vi "Main.vi"() -> ()   [LabVIEW 2014]
uses:
  QTMDriver 2013/CustomIO.ctl
  <vilib>/myRIO/Instrument Drivers/Onboard IO/AI/typedefs/AI Reference.ctl
  <vilib>/myRIO/Common/Instrument Driver Framework/Utilities/typedefs/myRIO Generic Hardware Reference.ctl
  <vilib>/myRIO/Common/Instrument Driver Framework/Utilities/typedefs/Hardware Version Enum.ctl
  <vilib>/myRIO/Common/Instrument Driver Framework/Utilities/typedefs/myRIO v1.0 Reference.ctl
  <vilib>/myRIO/Common/Instrument Driver Framework/Utilities/typedefs/Generic FPGA Reference.ctl
  <vilib>/myRIO/Common/Instrument Driver Framework/myRIO v1.0/AI/typedefs/AI Channels List.ctl
  <vilib>/myRIO/Common/Instrument Driver Framework/myRIO v1.0/AI/typedefs/AI Channels Enum.ctl
  <vilib>/myRIO/Common/Instrument Driver Framework/Utilities/typedefs/Analog Scaling Constants List.ctl
  <vilib>/myRIO/Common/Instrument Driver Framework/Utilities/typedefs/Analog Scaling Constants.ctl
  <vilib>/userdefined/High Color/nirio_resource_hc.ctl
  <vilib>/myRIO/Common/Instrument Driver Framework/Utilities/vis/Is FPGA Ref Available.vi
  <vilib>/myRIO/Common/Instrument Driver Framework/myRIO v1.0/AI/vis/myRIO v1.1 Open AI.vi
  <vilib>/myRIO/Instrument Drivers/Onboard IO/AI/vis/Read.vi
  <vilib>/myRIO/Common/Instrument Driver Framework/Utilities/vis/Validate Channels.vi
  <vilib>/myRIO/Common/Instrument Driver Framework/myRIO v1.0/AI/vis/myRIO v1.0 Reserve AI.vi
  <vilib>/myRIO/Common/Instrument Driver Framework/myRIO v1.0/UART/vis/myRIO v1.0 Close UART.vi
  <vilib>/myRIO/Common/Instrument Driver Framework/myRIO v1.0/AI/vis/myRIO v1.0 Build MUX Configuration AI.vi
  <vilib>/myRIO/Common/Instrument Driver Framework/myRIO v1.0/Resource Manager/vis/myRIO v1.0 Reserve Channel List.vi
  <vilib>/myRIO/Common/Instrument Driver Framework/myRIO v1.0/Resource Manager/vis/myRIO v1.0 Reserve Channel.vi
  <vilib>/myRIO/Common/Instrument Driver Framework/myRIO v1.0/Resource Manager/vis/myRIO v1.0 Unreserve Channel.vi
  <vilib>/myRIO/Common/Instrument Driver Framework/myRIO v1.0/Resource Manager/vis/myRIO v1.0 Build Mutex Name.vi
  <vilib>/Utility/VariantDataType/GetNumericInfo.vi
  <vilib>/Utility/error.llb/Error Cluster From Error Code.vi
  <vilib>/myRIO/Common/Instrument Driver Framework/myRIO v1.0/myRIO v1.1 Open.vi
  <vilib>/myRIO/Common/Instrument Driver Framework/myRIO v1.0/AI/vis/myRIO v1.0 Get Scaling Constants AI.vi
  <vilib>/myRIO/Common/Instrument Driver Framework/Utilities/vis/IO Manager.vi
  <vilib>/myRIO/Common/Instrument Driver Framework/Utilities/vis/Configuration Manager.vi
  <vilib>/myRIO/Common/Instrument Driver Framework/myRIO v1.0/myRIO v1.0 Close.vi
  <vilib>/myRIO/Common/Instrument Driver Framework/myRIO v1.0/AI/vis/myRIO v1.0 Read AI.vi
  <vilib>/myRIO/Common/Instrument Driver Framework/Utilities/vis/FPGA Ref Manager.vi
  <vilib>/myRIO/Common/Instrument Driver Framework/myRIO v1.0/myRIO v1.0 Reset FPGA.vi
  <vilib>/myRIO/Common/Instrument Driver Framework/myRIO v1.0/IRQ/vis/myRIO v1.0 IRQ Info FGV.vi
  <vilib>/myRIO/Common/Instrument Driver Framework/myRIO v1.0/IRQ/vis/myRIO v1.0 Timer IRQ Info FGV.vi
  <vilib>/myRIO/Common/Instrument Driver Framework/myRIO v1.0/IRQ/vis/myRIO v1.0 ISR Agent.vi
  <vilib>/myRIO/Express VI/Onboard IO/AI/AI Express VI.xnode
  <vilib>/myRIO/Instrument Drivers/Onboard IO/AI/vis/myRIO AI Open.xnode
  <vilib>/myRIO/Instrument Drivers/Utilities/Utilities.lvlib
  <vilib>/myRIO/Instrument Drivers/Onboard IO/AI/AI.lvlib
panel:
  out "p_d":dbl[](array[numeric])
  in  "psiplot 4":cluster{"psi_d":dbl, "psi":dbl}
  out "p_d":dbl[](array[numeric])
  out "wpPath":cluster{"x":dbl, "y":dbl}[](array[cluster])
  out "iOut WPDP":dbl
  out "psiplot WPDP":cluster{"Double":dbl, "y_r":dbl, "y":dbl}(graph)
  out "yplot WPDP":cluster{"Double":dbl, "y_r":dbl, "y":dbl}(graph)
  out "xplot WPDP":cluster{"Double":dbl, "y_r":dbl, "y":dbl}(graph)
  out "WithinProximity WPDP":bool
  out "e_psi 2":dbl
  out "45degrees":bool
  out "iOut":dbl
  out "e_psi":dbl
  out "proximity straight":dbl
  out "plotpsi str":cluster{"psi_d":dbl, "psi":dbl}(graph)
  out "psiplot str":cluster{"psi_d":dbl, "psi":dbl}
  in  "u":dbl[](array[numeric])
  out "plotdelta":dbl(graph)
  out "plotpsi":cluster{"psi_d":dbl, "psi":dbl}(graph)
  out "WithinProximity radius":bool
  out "proximity":dbl
  out "psiplot 3":cluster{"psi_d":dbl, "psi":dbl}
  out "psiplot 2":cluster{"e_d":dbl, "e_r":dbl, "psi":dbl}
  out "yplot 2":cluster{"y_d":dbl, "y_r":dbl, "y":dbl}
  out "xplot 2":cluster{"x_d":dbl, "x_r":dbl, "x":dbl}
  out "psiplot":cluster{"Double":dbl, "y_r":dbl, "y":dbl}(graph)
  out "yplot":cluster{"Double":dbl, "y_r":dbl, "y":dbl}(graph)
  out "xplot":cluster{"Double":dbl, "y_r":dbl, "y":dbl}(graph)
  out "straightPath":cluster{"x":dbl, "y":dbl}[](array[cluster])
  out "ellipsePath":cluster{"x":dbl, "y":dbl}[](array[cluster])
  out "y":dbl
  out "x":dbl
  out "B/AI2 (Pin 7)":dbl
  in  "stop":bool
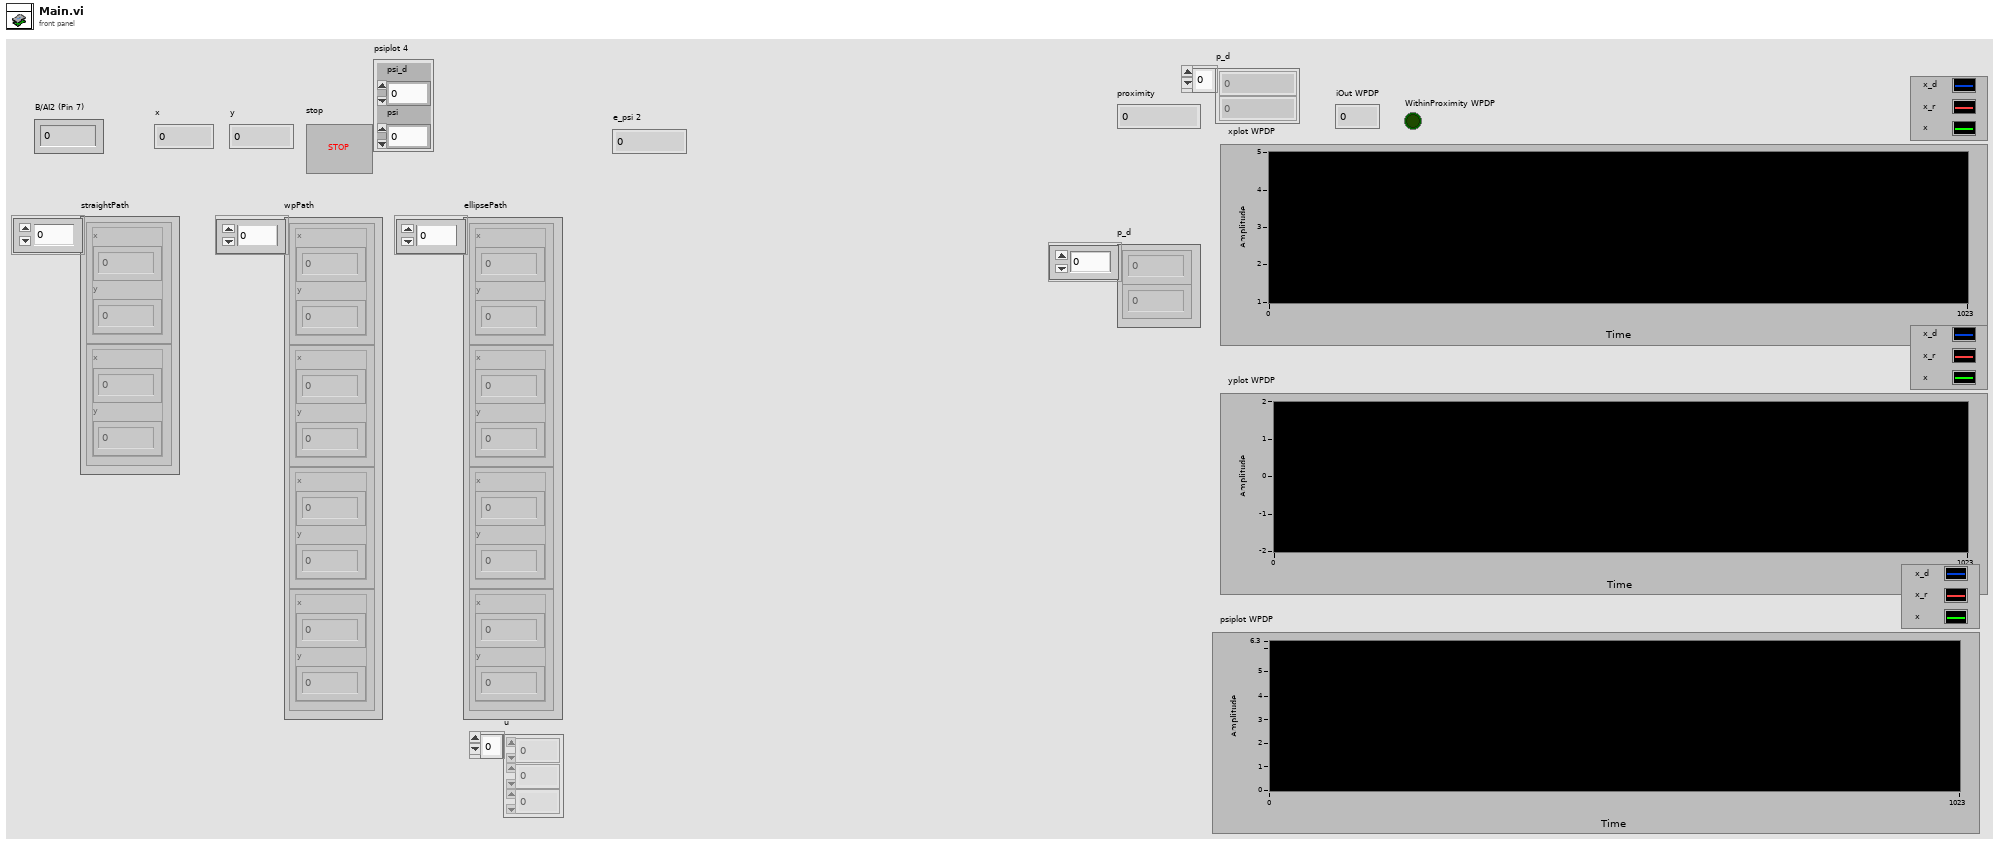
[diagram p1: front panel]
types:
  T1 = typedef "CustomIO.ctl" = enum16{"Init", "Read", "Write", "Close", "N/O"}
  T2 = typedef "AI.lvlib/AI Reference.ctl" = cluster{"myRIO Reference":T3, "AI Channels List":T7, "AI Scaling Constants List":T9}
  T3 = typedef "myRIO Generic Hardware Reference.ctl" = cluster{"myRIO Model":T4, "myRIO Hardware Reference":T5}
  T4 = typedef "Hardware Version Enum.ctl" = enum16{"Unknown", "myRIO-1900", "myRIO-1950"}
  T5 = typedef "myRIO v1.0 Reference.ctl" = cluster{"Generic FPGA Reference":T6, "Allow multiple opens":bool}
  T6 = typedef "Generic FPGA Reference.ctl" = refnum<k20>
  T7 = typedef "AI Channels List.ctl" = T8[]
  T8 = typedef "AI Channels Enum.ctl" = enum16{"Not Connected", "AudioIn/Left", "AudioIn/Right", "C/AI0", "C/AI1", "A/AI0", "A/AI1", "A/AI2", "A/AI3", "B/AI0", "B/AI1", "B/AI2", "B/AI3"}
  T9 = typedef "Analog Scaling Constants List.ctl" = T10[]
  T10 = typedef "Analog Scaling Constants.ctl" = cluster{"LSB Weight (Volts)":dbl, "Offset (Volts)":dbl, "Signed?":bool}
  T11 = typedef "nirio_resource_hc.ctl" = tag
  T12 = cluster{"proportional gain (Kc)":dbl, "integral time (Ti, min)":dbl, "derivative time (Td, min)":dbl}
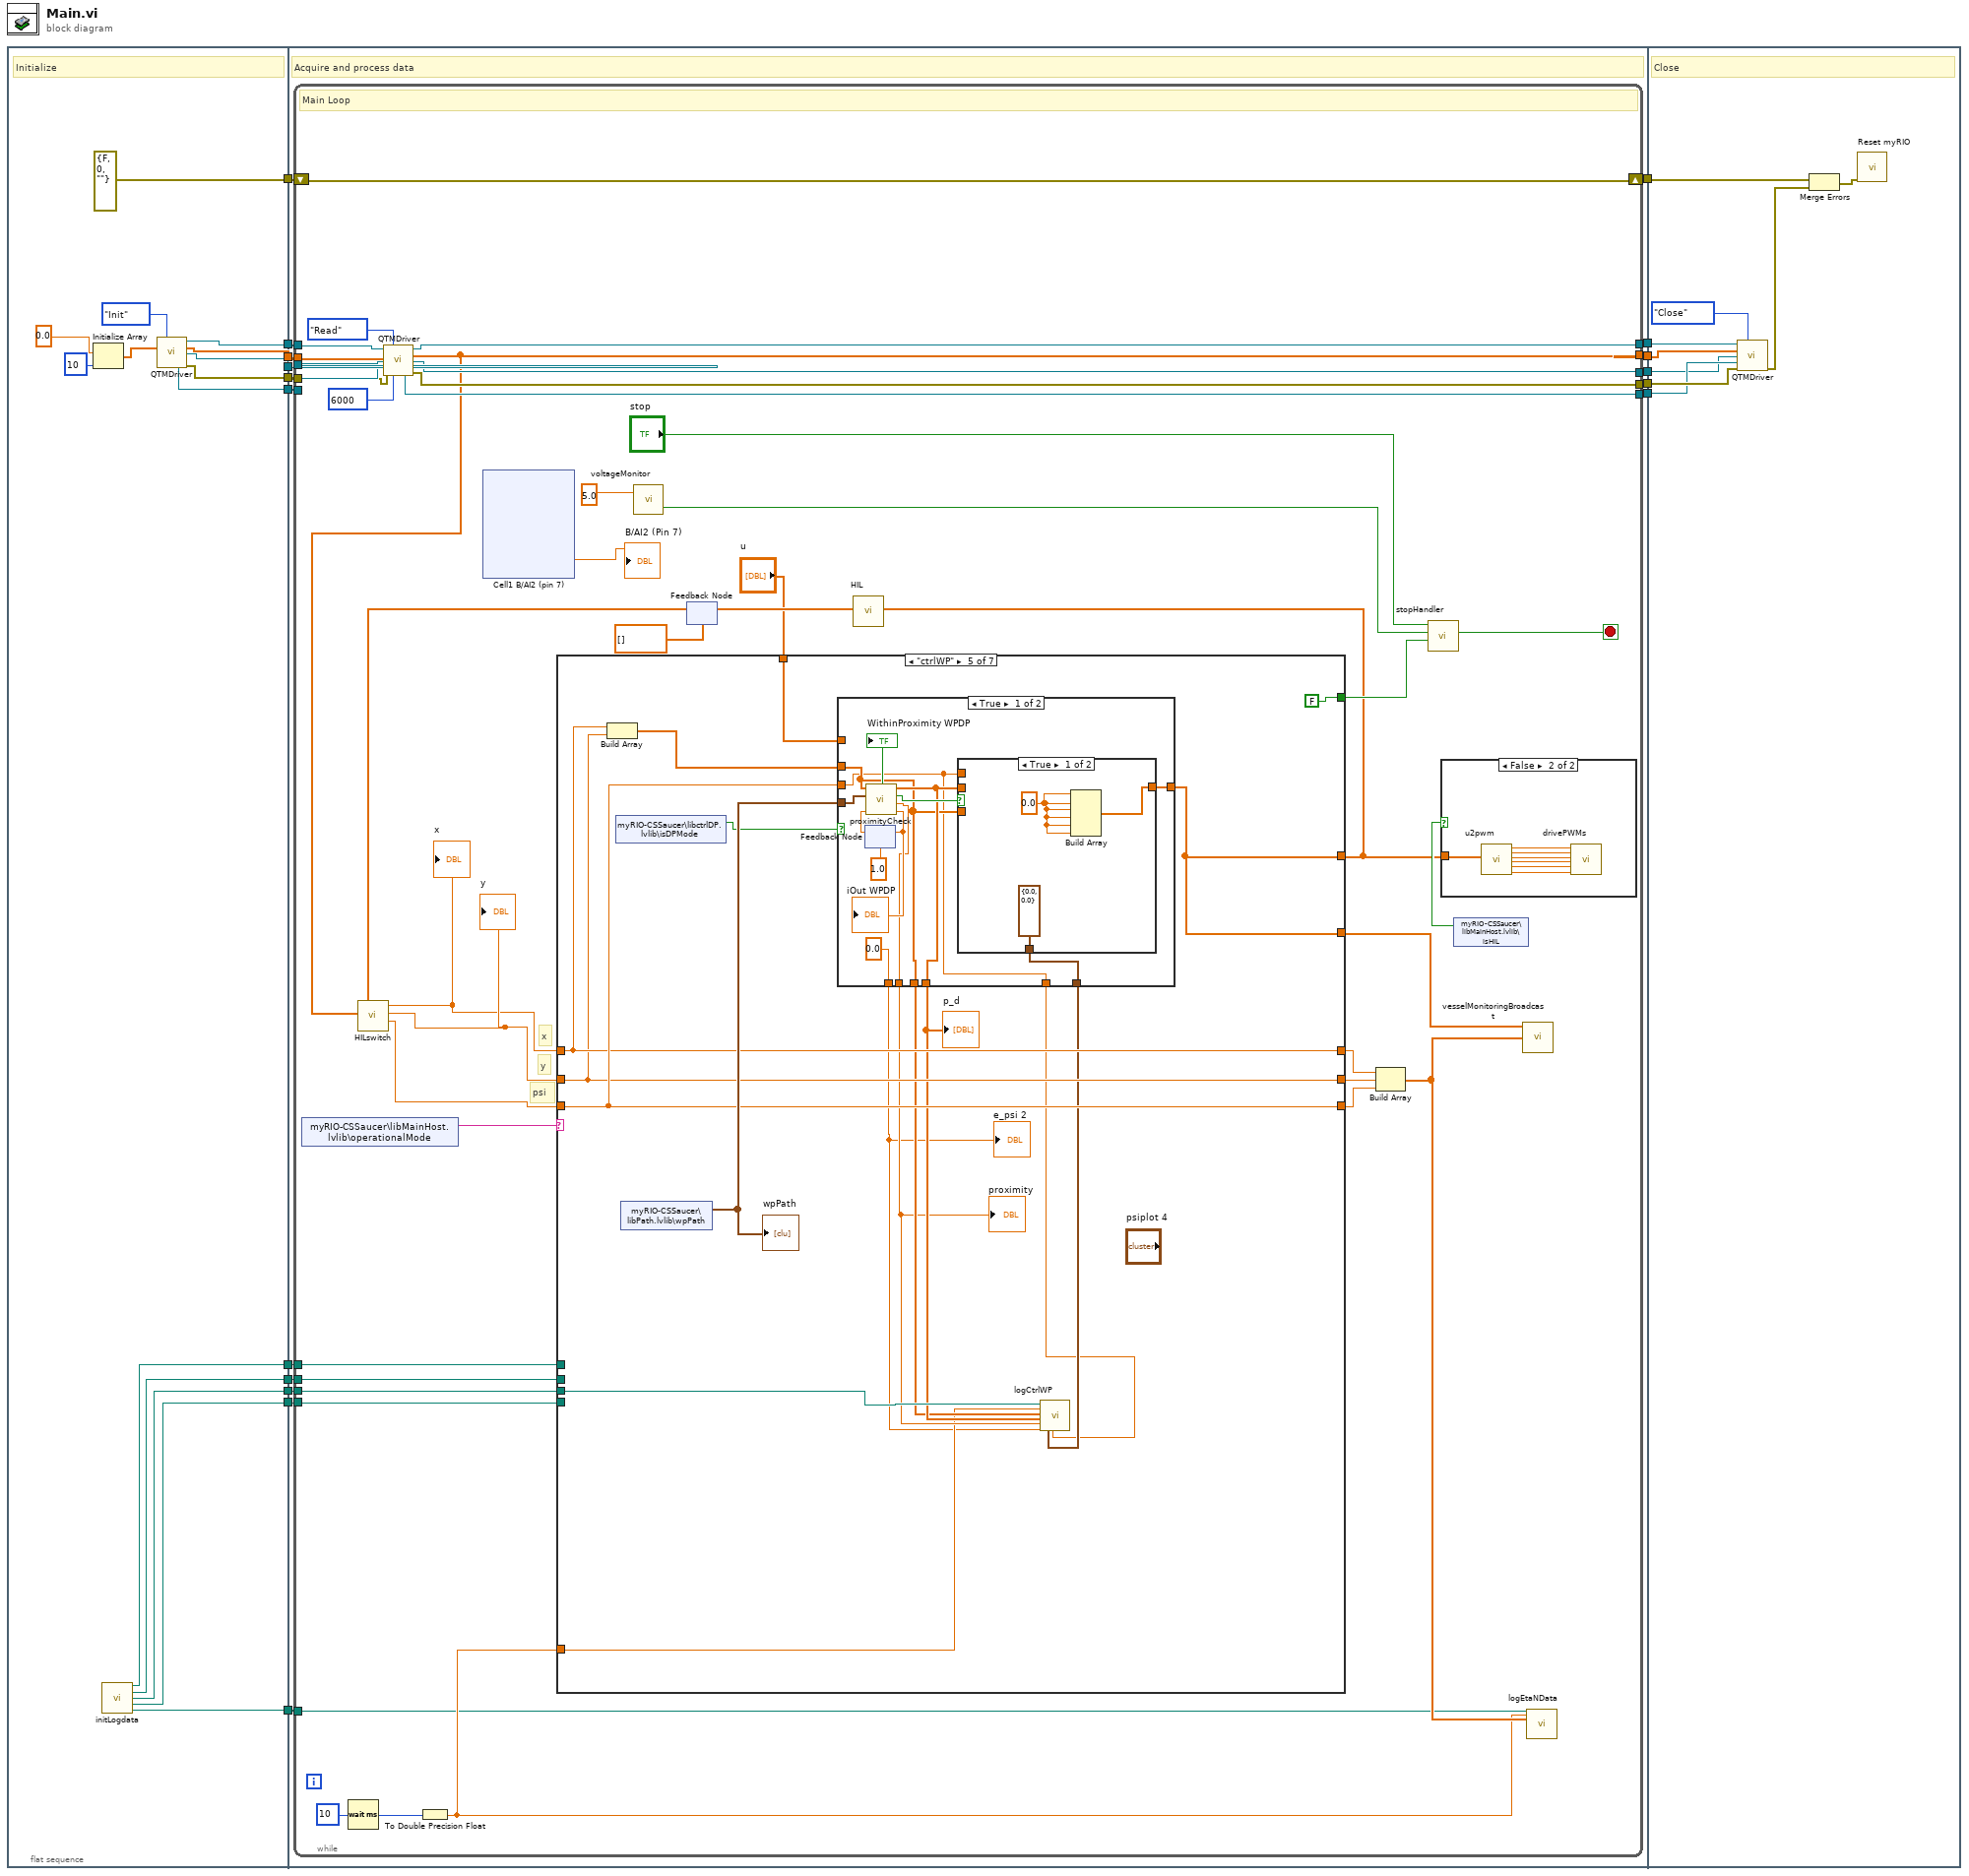
[diagram p0: block diagram]
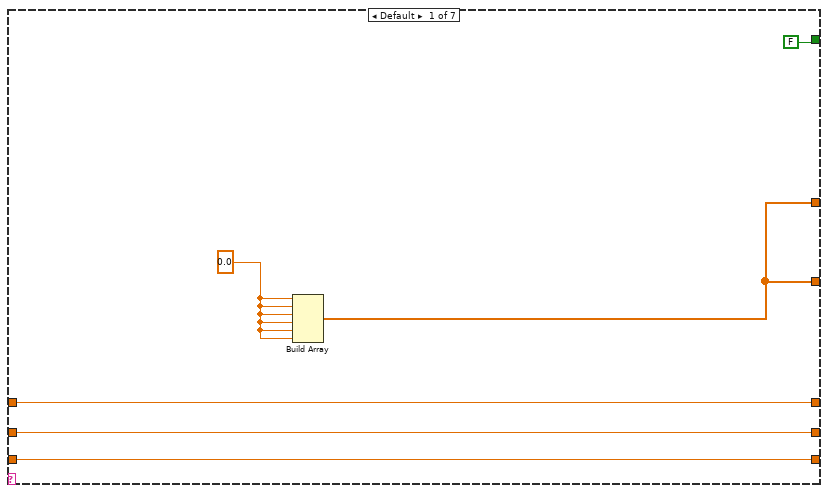
[diagram p3: hidden frame]
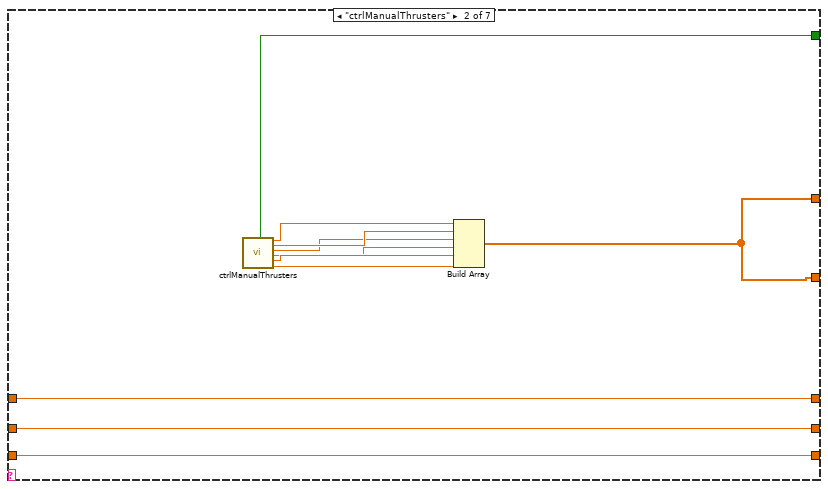
[diagram p4: hidden frame]
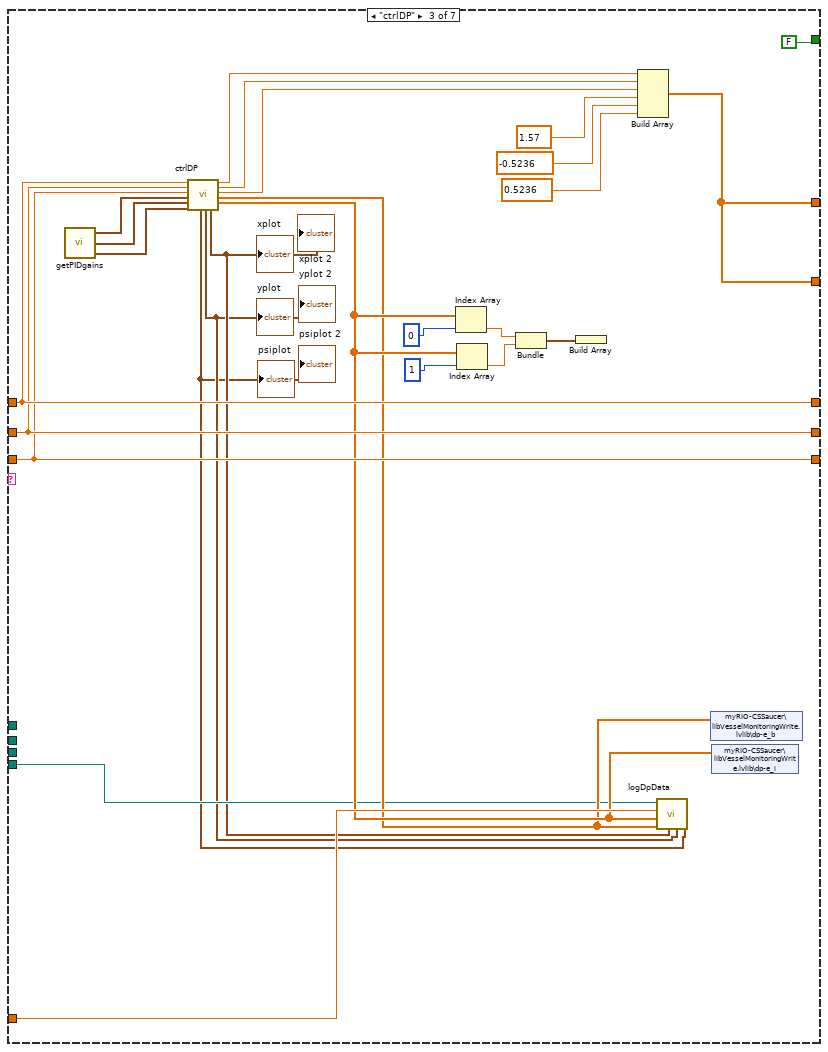
[diagram p5: hidden frame]
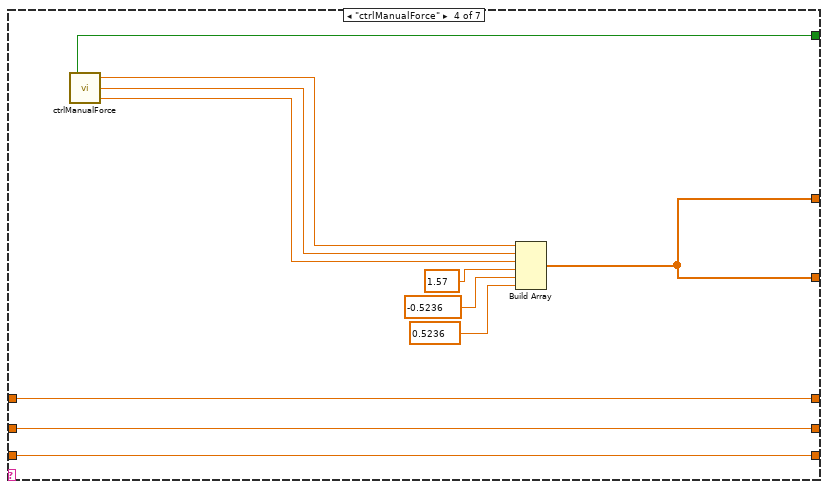
[diagram p6: hidden frame]
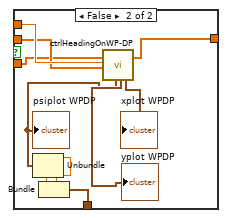
[diagram p7: hidden frame]
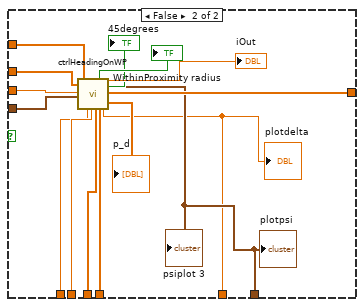
[diagram p8: hidden frame]
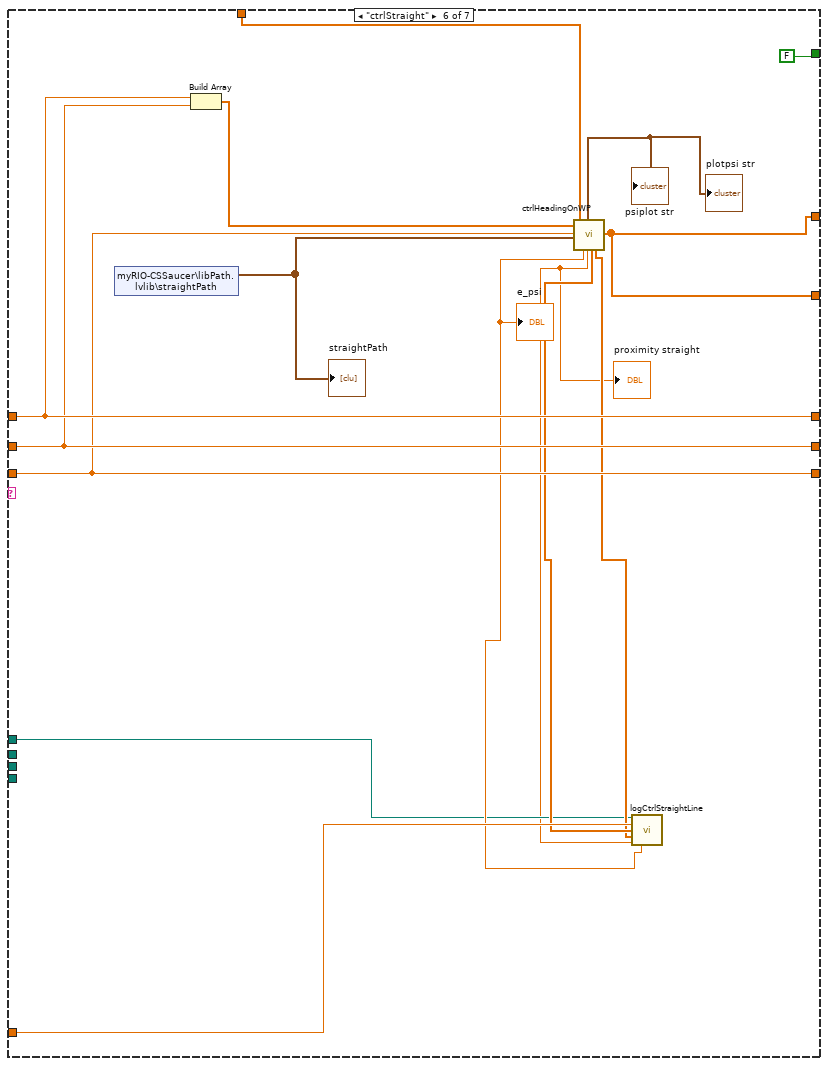
[diagram p9: hidden frame]
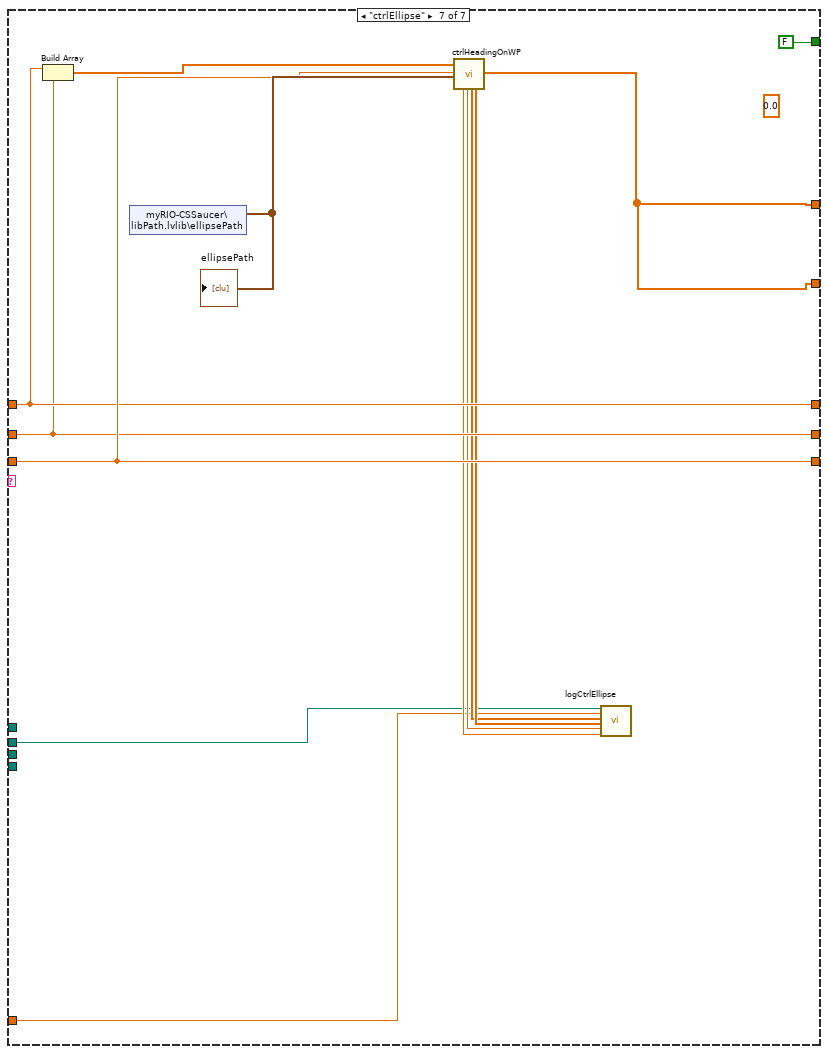
[diagram p10: hidden frame]
diagram:
  n1 = flat-sequence {
    tunnel: [errorcluster {"status"=FALSE, "code"=0, "source"=""} ("error out")] -> w17
    tunnel: [w26] -> w15
    tunnel: [w27] -> w14
    tunnel: [w25] -> w13
    tunnel: [w24] -> w12
    tunnel: [w23] -> w11
    tunnel: [w18] -> w5
    tunnel: [w22] -> w4
    tunnel: [w21] -> w3
    tunnel: [w20] -> w2
    tunnel: [w19] -> w1
    tunnel: w17 -> [w49]
    tunnel: [w48] -> w16
    tunnel: w15 -> [w47]
    tunnel: w14 -> [w46]
    tunnel: w13 -> [w45]
    tunnel: w12 -> [w44]
    tunnel: w11 -> [w43]
    tunnel: [w42] -> w10
    tunnel: [w41] -> w9
    tunnel: [w40] -> w8
    tunnel: [w39] -> w7
    tunnel: [w38] -> w6
    tunnel: w5 -> [w37]
    tunnel: w4 -> [w36]
    tunnel: w3 -> [w35]
    tunnel: w2 -> [w34]
    tunnel: w1 -> [w33]
    tunnel: w16 -> [w276]
    tunnel: w10 -> [w278]
    tunnel: w9 -> [w279]
    tunnel: w8 -> [w280]
    tunnel: w7 -> [w282]
    tunnel: w6 -> [w281]
    frame #0 {
      # "Initialize"
      n2 = Initialize Array(0.0, 10 ("dimension size")) -> (w28:dbl[])
      n3 = call "initLogdata.vi"() -> ("straightPath"=w22:path, "ellipsePath"=w21:path, "wpPath"=w20:path, "dpPath"=w19:path, "eta_iPath"=w18:path)  [unwired: 11 in]
      n4 = call "QTMDriver.vi"("Ring"=CustomIO."Init", "DataIn"=w28) -> ("connection ID out"=w26:refnum<k5>, "DataOut"=w27:dbl[], "QTMqueue Out"=w25:refnum<queue>, "VI Refnum QTMTask Out"=w23:refnum<vi>, "error out"=w24:errorcluster)  [unwired: 7 in, 2 out]
    }
    frame #1 {
      # "Acquire and process data"
      n5 = while {
        shift-right: [w69] -> w48
        shift-left: w49 -> [w69]
        tunnel: w47 -> [w90]
        tunnel: w46 -> [w89]
        tunnel: w45 -> [w88]
        tunnel: w44 -> [w86]
        tunnel: w43 -> [w87]
        tunnel: [w82] -> w42
        tunnel: [w64] -> w41
        tunnel: [w83] -> w40
        tunnel: [w84] -> w39
        tunnel: [w81] -> w38
        tunnel: w37 -> [w70]
        tunnel: w36 -> [w71]
        tunnel: w35 -> [w57]
        tunnel: w34 -> [w56]
        tunnel: w33 -> [w55]
        stop <- w65 stop-if-true
        # "x"
        # "y"
        # "psi"
        # "Main Loop"
        n6 = shared-variable "myRIO-CSSaucer\\libMainHost.lvlib\\operationalMode"() -> (w80:string)  [unwired: 1 in, 1 out]
        n7 = Wait (ms)(milliseconds to wait=u32 10) -> (millisecond timer value=w78:u32)
        n8 = call "QTMDriver.vi"("connection ID"=w90, "Ring"=CustomIO."Read", "DataIn"=w89, "QTMqueue"=w88, "VI Refnum QTMTask"=w87, "error in"=w86, "timeout ms (25000)"=6000) -> ("connection ID out"=w82:refnum<k5>, "DataOut"=w64:dbl[], "QTMqueue Out"=w83:refnum<queue>, "VI Refnum QTMTask Out"=w81:refnum<vi>, "error out"=w84:errorcluster)  [unwired: 2 in, 2 out]
        n9 = To Double Precision Float(number=w78) -> (double precision float=w72:dbl)
        n10 = xnode "Cell1 B/AI2 (pin 7)"() -> ("B/AI2 (Pin 7)"=→"B/AI2 (Pin 7)":dbl)  [unwired: 1 in, 1 out]
        n11 = call "voltageMonitor.vi"("Cell 1 voltage"=5.0) -> ("Boolean"=w68:bool)  [unwired: 2 in]
        n12 = feedback #1(dbl[] [] ("U")) -> (w63:dbl[])
        n13 = call "HILswitch.vi"("u_HIL"=w63, "QTM"=w64) -> ("psi"=w61:dbl, "y"=w60:dbl, "x"=w59:dbl)  [unwired: 7 in]
        "x" <- w59
        "y" <- w60
        n14 = case shown="\"ctrlWP\"" w80 {
          tunnel: [w99 w111 w120 w142 w163 w213 w231] -> w54
          tunnel: [w104 w115 w136 w148 w168 w220 w235] -> w74
          tunnel: [w103 w114 w138 w149 w167 w222 w234] -> w75
          tunnel: [w99 w111 w120 w142 w163 w213 w231] -> w79
          tunnel: w59 -> [w103 w114 w138 w149 w167 w222 w234]
          tunnel: w61 -> [w104 w115 w136 w148 w168 w220 w235]
          tunnel: [w102 w113 w137 w147 w166 w221 w233] -> w76
          tunnel: w60 -> [w102 w113 w137 w147 w166 w221 w233]
          tunnel: w72 -> [_ _ w127 _ w158 w218 w226]
          tunnel: w71 -> [_ _ _ _ _ w214 _]
          tunnel: [FALSE w112 FALSE w146 FALSE FALSE FALSE] -> w67
          tunnel: w57 -> [_ _ _ _ _ _ w225]
          tunnel: w56 -> [_ _ _ _ w162 _ _]
          tunnel: w55 -> [_ _ w119 _ _ _ _]
          tunnel: "u" -> [_ _ _ _ w157 w212 _]
          frame Default {
            w100 = 0.0
            n15 = Build Array(w100, w100, w100, w100, w100, w100) -> (w99:dbl[])
          }
          frame "ctrlManualThrusters" {
            n16 = call "ctrlManualThrusters.vi"() -> ("stop"=w112:bool, "u_t0"=w108:dbl, "u_t1"=w110:dbl, "u_t2"=w106:dbl, "alpha_t0"=w107:dbl, "alpha_t1"=w109:dbl, "alpha_t2"=w105:dbl)  [unwired: 13 in]
            n17 = Build Array(w108, w110, w106, w107, w109, w105) -> (w111:dbl[])
          }
          frame "ctrlDP" {
            n18 = call "getPIDgains.vi"() -> ("PID psi"=w133:T12, "PID y"=w134:T12, "PID x"=w135:T12)  [unwired: 3 in]
            n19 = call "ctrlDP.vi"("x"=w138, "y"=w137, "psi"=w136, "PID 0"=w135, "PID 1"=w134, "PID 2"=w133) -> ("psiplot"=w116:cluster{"Double":dbl, "y_r":dbl, "y":dbl}, "yplot"=w117:cluster{"Double":dbl, "y_r":dbl, "y":dbl}, "xplot"=w118:cluster{"Double":dbl, "y_r":dbl, "y":dbl}, "u_0"=w123:dbl, "u_1"=w122:dbl, "u_2"=w121:dbl, "eta_e_n"=w125:dbl[], "eta_e_b"=w126:dbl[])  [unwired: 6 in]
            "xplot" <- w118
            "yplot" <- w117
            "psiplot" <- w116
            "xplot 2" <- w118
            "yplot 2" <- w117
            "psiplot 2" <- w116
            n20 = Index Array(array=w126, index=0) -> (element=w128:dbl)
            n21 = Index Array(array=w126, index=1) -> (element=w129:dbl)
            n22 = Bundle(w128, w129) -> (w132:cluster{dbl, dbl})  [unwired: 1 in]
            n23 = Build Array(w132) -> ()  [unwired: 1 out]
            n24 = Build Array(w123, w122, w121, 1.57 ("element"), -0.5236 ("element"), 0.5236 ("element")) -> (w120:dbl[])
            n25 = call "logDpData.vi"("psiplot"=w116, "yplot"=w117, "xplot"=w118, "e_i"=w125, "e_b"=w126, "time"=w127, "dpPath"=w119) -> ()  [unwired: 5 in]
            n26 = shared-variable "myRIO-CSSaucer\\libVesselMonitoringWrite.lvlib\\dp-e_b"(w125) -> ()  [unwired: 1 in, 1 out]
            n27 = shared-variable "myRIO-CSSaucer\\libVesselMonitoringWrite.lvlib\\dp-e_i"(w126) -> ()  [unwired: 1 in, 1 out]
          }
          frame "ctrlManualForce" {
            n28 = call "ctrlManualForce.vi"() -> ("u_2"=w143:dbl, "u_1"=w144:dbl, "u_0"=w145:dbl, "stopManualForce_DSH"=w146:bool)  [unwired: 2 in]
            n29 = Build Array(w145, w144, w143, 1.57 ("element"), -0.5236 ("element"), 0.5236 ("element")) -> (w142:dbl[])
          }
          frame "ctrlWP" {
            n30 = Build Array(w167, w166) -> (w165:dbl[])
            n31 = shared-variable "myRIO-CSSaucer\\libctrlDP.lvlib\\isDPMode"() -> (w155:bool)  [unwired: 1 in, 1 out]
            n32 = shared-variable "myRIO-CSSaucer\\libPath.lvlib\\wpPath"() -> (w169:cluster{"x":dbl, "y":dbl}[])  [unwired: 1 in, 1 out]
            "wpPath" <- w169
            n33 = case shown="True" w155 {
              tunnel: w169 -> [w181 w209]
              tunnel: w168 -> [w171 w208]
              tunnel: w165 -> [w172 w207]
              tunnel: [w182 w206] -> w163
              tunnel: [w175 w205] -> w161
              tunnel: [w172 w204] -> w160
              tunnel: [w176 w203] -> w159
              tunnel: w157 -> [_ w201]
              tunnel: [0.0 w198] -> w156
              tunnel: [w170 w197] -> w154
              tunnel: [w171 w196] -> w153
              frame True {
                n34 = feedback #2(1.0) -> (w177:dbl)
                n35 = call "proximityCheck.vi"("i"=w177, "pathCoords"=w181, "p(t)"=w172) -> ("iOut"=w178:dbl, "e"=w176:dbl, "indexOutOfBounds"=w180:bool, "p_d"=w175:dbl[], "WithinProximity radius"=→"WithinProximity WPDP":bool)  [unwired: 1 in]
                "iOut WPDP" <- w178
                n36 = feedback-in #2(w178) -> ()
                n37 = case shown="True" w180 {
                  tunnel: [w184 w195] -> w182
                  tunnel: w171 -> [_ w194]
                  tunnel: w175 -> [_ w191]
                  tunnel: w172 -> [_ w190]
                  tunnel: [cluster{"Double":dbl, "y":dbl} {"Double"=0.0, "y"=0.0} w186] -> w170
                  frame True {
                    w185 = 0.0
                    n38 = Build Array(w185, w185, w185, w185, w185, w185) -> (w184:dbl[])
                  }
                  frame False {
                    n39 = call "ctrlHeadingOnWP-DP.vi"("p(t)"=w190, "psi"=w194, "p_d"=w191) -> ("psiplot"=w189:cluster{"Double":dbl, "y_r":dbl, "y":dbl}, "yplot"=→"yplot WPDP":cluster{"Double":dbl, "y_r":dbl, "y":dbl}, "xplot"=→"xplot WPDP":cluster{"Double":dbl, "y_r":dbl, "y":dbl}, "U"=w195:dbl[])  [unwired: 11 in, 2 out]
                    "psiplot WPDP" <- w189
                    n40 = Unbundle(w189) -> ("Double"=w188:dbl, "y"=w187:dbl)  [unwired: 1 out]
                    n41 = Bundle("Double"=w188, "y"=w187) -> (w186:cluster{"Double":dbl, "y":dbl})  [unwired: 1 in]
                  }
                }
              }
              frame False {
                n42 = call "ctrlHeadingOnWP.vi"("p(t)"=w207, "psi"=w208, "pathCoords"=w209, "u"=w201) -> ("45degrees"=→"45degrees":bool, "e_psi"=w198:dbl, "psiplot"=w197:cluster{"psi_d":dbl, "psi":dbl}, "e"=w203:dbl, "eta_i 2"=w204:dbl[], "WithinProximity radius"=→"WithinProximity radius":bool, "eta_r"=w205:dbl[], "delta"=w196:dbl, "iOut"=→"iOut":dbl, "U"=w206:dbl[])  [unwired: 14 in]
                "psiplot 3" <- w197
                "plotpsi" <- w197
                "plotdelta" <- w196
                "p_d" <- w205
              }
            }
            "proximity" <- w159
            "e_psi 2" <- w156
            "p_d" <- w161
            n43 = call "logCtrlWP.vi"("wpPath"=w162, "time"=w158, "eta_i"=w160, "eta_r"=w161, "e_i"=w159, "e_psi"=w156, "psiplot"=w154, "delta"=w153) -> ()  [unwired: 12 in]
          }
          frame "ctrlStraight" {
            n44 = shared-variable "myRIO-CSSaucer\\libPath.lvlib\\straightPath"() -> (w224:cluster{"x":dbl, "y":dbl}[])  [unwired: 1 in, 1 out]
            "straightPath" <- w224
            n45 = Build Array(w222, w221) -> (w223:dbl[])
            n46 = call "ctrlHeadingOnWP.vi"("p(t)"=w223, "psi"=w220, "pathCoords"=w224, "u"=w212) -> ("e_psi"=w215:dbl, "psiplot"=→"psiplot str" →"plotpsi str":cluster{"psi_d":dbl, "psi":dbl}, "e"=w211:dbl, "eta_i 2"=w217:dbl[], "eta_r"=w216:dbl[], "U"=w213:dbl[])  [unwired: 14 in, 4 out]
            "proximity straight" <- w211
            "e_psi" <- w215
            n47 = call "logCtrlStraightLine.vi"("straightPath"=w214, "time"=w218, "eta_i"=w217, "eta_r"=w216, "e_i"=w211, "e_psi"=w215) -> ()  [unwired: 10 in]
          }
          frame "ctrlEllipse" {
            (unwired) 0.0
            n48 = Build Array(w234, w233) -> (w232:dbl[])
            n49 = shared-variable "myRIO-CSSaucer\\libPath.lvlib\\ellipsePath"() -> (w236:cluster{"x":dbl, "y":dbl}[])  [unwired: 1 in, 1 out]
            "ellipsePath" <- w236
            n50 = call "ctrlHeadingOnWP.vi"("p(t)"=w232, "psi"=w235, "pathCoords"=w236) -> ("e_psi"=w229:dbl, "e"=w228:dbl, "eta_i 2"=w227:dbl[], "eta_r"=w230:dbl[], "U"=w231:dbl[])  [unwired: 15 in, 5 out]
            n51 = call "logCtrlEllipse.vi"("EllipsePath"=w225, "time"=w226, "eta_i"=w227, "eta_r"=w230, "e_i"=w228, "e_psi"=w229) -> ()  [unwired: 14 in]
          }
        }
        n52 = call "HIL.vi"("U"=w54) -> ("eta"=w53:dbl[])  [unwired: 10 in]
        n53 = feedback-in #1(w53) -> ()
        n54 = Build Array(w75, w76, w74) -> (w73:dbl[])
        n55 = call "stopHandler.vi"("stopOperationalMode"=w67, "stopVoltageAlert"=w68, "stopMain"="stop") -> ("stop"=w65:bool)  [unwired: 8 in]
        n56 = shared-variable "myRIO-CSSaucer\\libMainHost.lvlib\\isHIL"() -> (w58:bool)  [unwired: 1 in, 1 out]
        n57 = case shown="False" w58 {
          tunnel: w54 -> [_ w92]
          frame True {
          }
          frame False {
            n58 = call "u2pwm.vi"("U"=w92) -> ("dc_u_t 0"=w98:dbl, "dc_u_t 1"=w97:dbl, "dc_u_t 2"=w96:dbl, "dc_rotation_t 0"=w95:dbl, "dc_rotation_t 1"=w94:dbl, "dc_rotation_t 2"=w93:dbl)  [unwired: 13 in]
            n59 = call "drivePWMs.vi"("u_t 0"=w98, "u_t 1"=w97, "u_t 2"=w96, "alpha 0"=w95, "alpha 1"=w94, "alpha 2"=w93) -> ()  [unwired: 14 in]
          }
        }
        n60 = call "vesselMonitoringBroadcast.vi"("U"=w79, "eta"=w73) -> ()  [unwired: 14 in]
        n61 = call "logEtaNData.vi"("eta_iPath"=w70, "time"=w72, "eta"=w73) -> ()  [unwired: 25 in]
      }
    }
    frame #2 {
      # "Close"
      n62 = call "QTMDriver.vi"("connection ID"=w278, "Ring"=CustomIO."Close", "DataIn"=w279, "QTMqueue"=w280, "VI Refnum QTMTask"=w281, "error in"=w282) -> ("error out"=w275:errorcluster)  [unwired: 3 in, 6 out]
      n63 = Merge Errors(w276, w275) -> (w277:errorcluster)
      n64 = call <vilib>:"Reset myRIO.vi"("error in (no error)"=w277) -> ()  [unwired: 10 in, 1 out]
    }
  }
